vi "checkout.vi"(7 "locked by?":string, 8 "error in (no error)":errorcluster) -> (0 "error out":errorcluster, 3 "GenericMicroscope out":refnum<class "GenericInstrument.lvclass">)   [LabVIEW 2010, in "GenericInstrument.lvclass"]
uses:
  GenericInstrument.lvclass
  class_data.vi
  common/classes/GenericComponent/GenericComponent/GenericComponent.lvclass
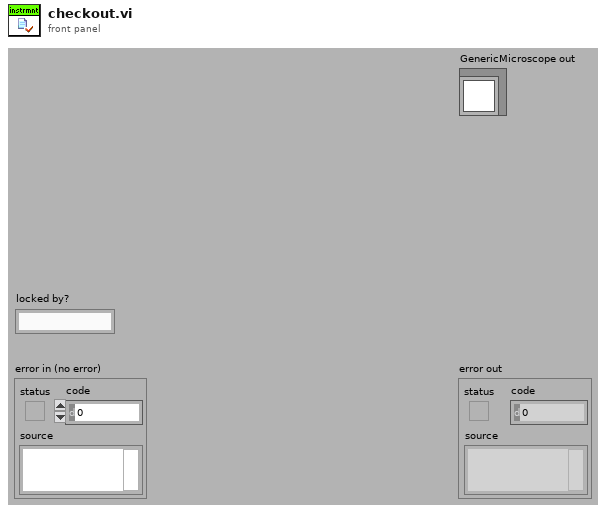
[diagram p1: front panel]
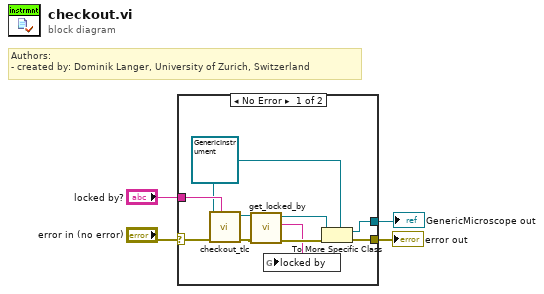
[diagram p0: block diagram]
diagram:
  # "Authors: \n- created by: Dominik Langer, University of Zurich, Switzerland"
  n1 = case shown="No Error" "error in (no error)" {
    selector: "error in (no error)" -> [w6 w15]
    tunnel: [w13 w15] -> w2
    tunnel: "locked by?" -> [w14 _]
    tunnel: [w12 _] -> w1
    frame No Error {
      w5 = refnum<class "GenericInstrument.lvclass"> refnum ("GenericMicroscope.lvclass")
      n2 = call-dynamic "checkout_tlc.vi"("locked by?"=w14, "error in (no error)"=w6, "GenericToplevelComponent in"=w5) -> ("error out"=w11:errorcluster, "GenericToplevelComponent out"=w10:refnum<class "GenericToplevelComponent.lvclass">)  [unwired: 7 in]
      n3 = call "get_locked_by.vi"("error in (no error)"=w11, "GenericPlugin.lvclass in"=w10) -> ("error out"=w9:errorcluster, "locked by"=w7:string, "GenericPlugin.lvclass out"=w8:refnum<class "GenericToplevelComponent.lvclass">)  [unwired: 7 out]
      n4 = global write "class_data.vi" "locked by"(w7) -> ()
      n5 = To More Specific Class(target class=w5, reference=w8, error in=w9) -> (specific class reference=w12:refnum<class "GenericInstrument.lvclass">, error out=w13:errorcluster)
    }
    frame Error {
    }
  }
  "error out" <- w2
  "GenericMicroscope out" <- w1
